vi "display_michelle_visjitter_adj.vi"() -> ()   [LabVIEW 2019]
uses:
  <vilib>/Analysis/Matrix/Datatypes/RealMatrix.ctl
  <vilib>/Utility/file.llb/Write Delimited Spreadsheet (DBL).vi
  <vilib>/Analysis/Matrix/NI_Matrix.lvlib
panel:
  in  "Stop":bool
  out "Num trials":u32=204
  out "ISI Time":dbl
  out "Stim TS":dbl
  out "Output":dbl[][](array[numeric])
  out "Output frame":T1
  out "Array temp1":T1
  out "Elapsed Time":dbl
  out "Display":bool=TRUE
  out "Trial":u32=1
  out "reward":dbl[](array[numeric])
  out "stim_id":dbl[](array[numeric])
  out "stim_loaded":dbl
  out "Timings":dbl[](array[numeric])
  out "Stimuli Loaded?":bool
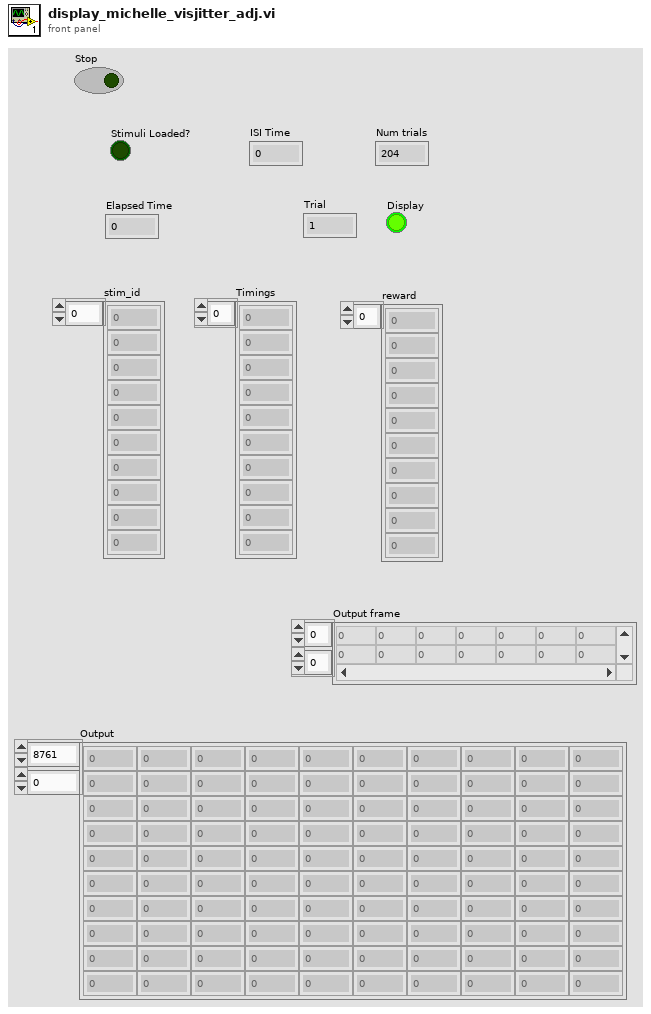
[diagram p1: front panel]
types:
  T1 = typedef "NI_Matrix.lvlib/RealMatrix.ctl" = dbl[][]
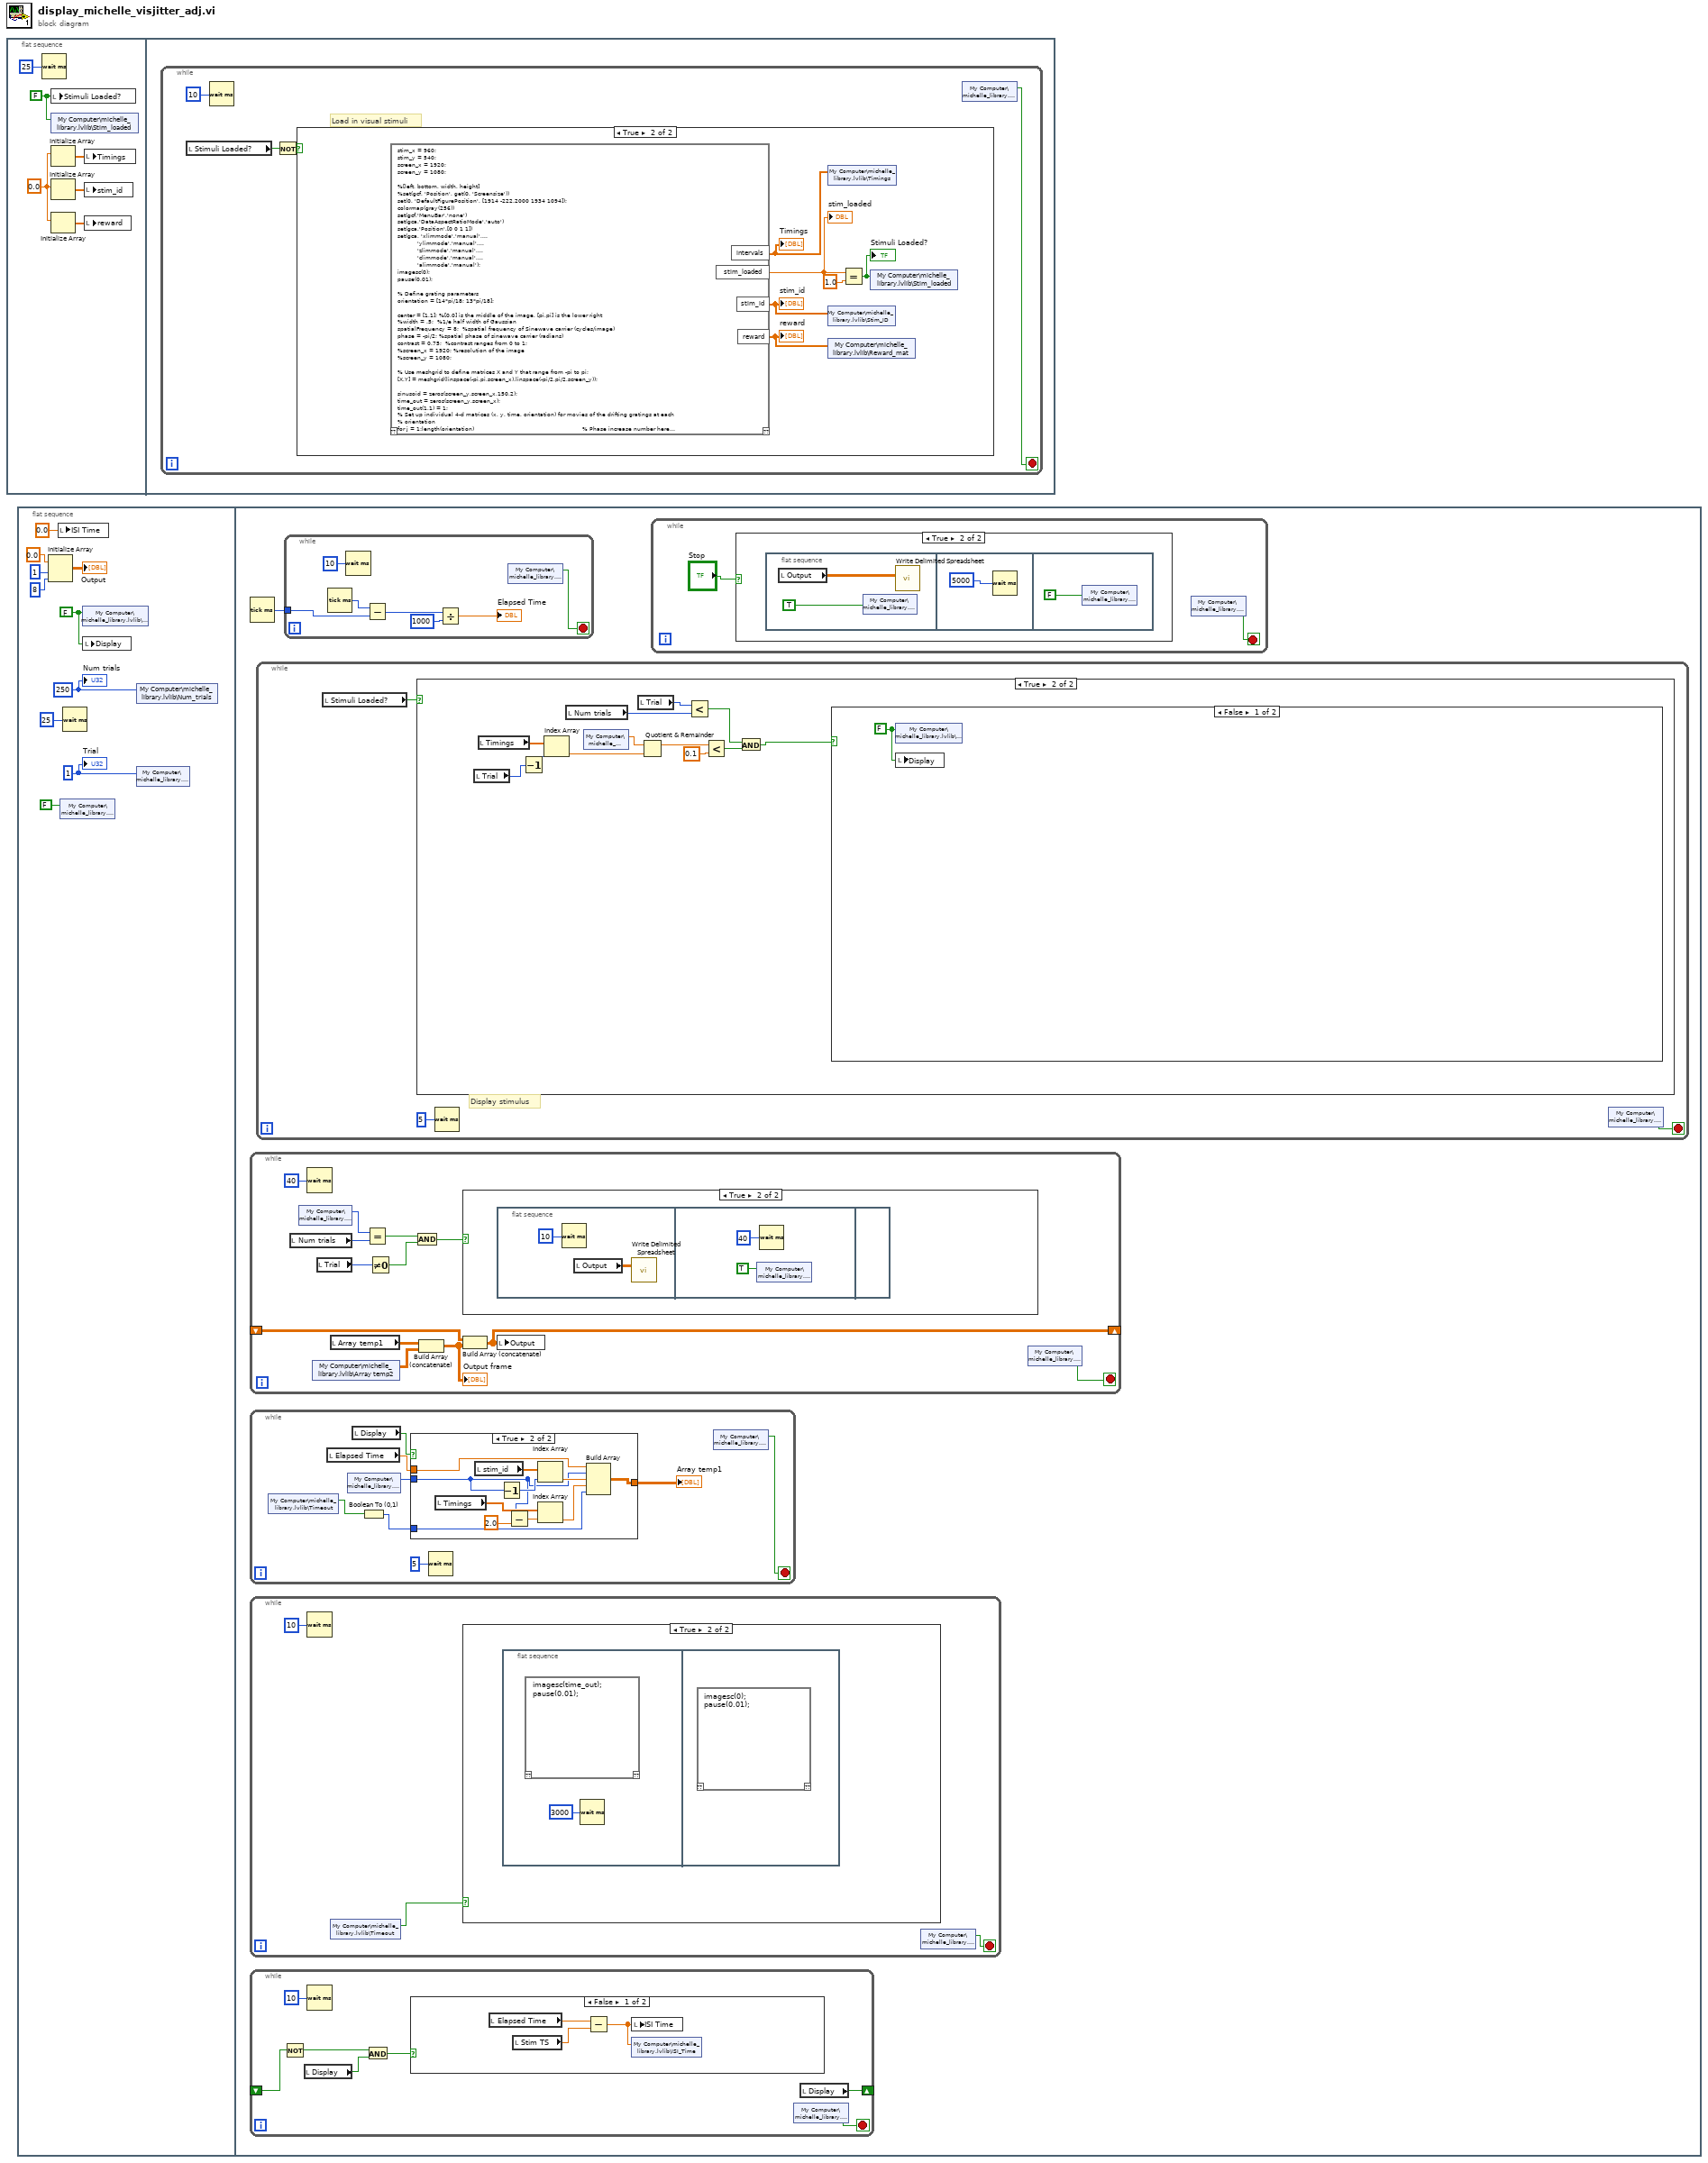
[diagram p0: block diagram]
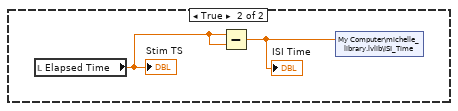
[diagram p5: hidden frame]
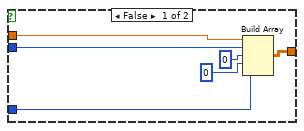
[diagram p6: hidden frame]
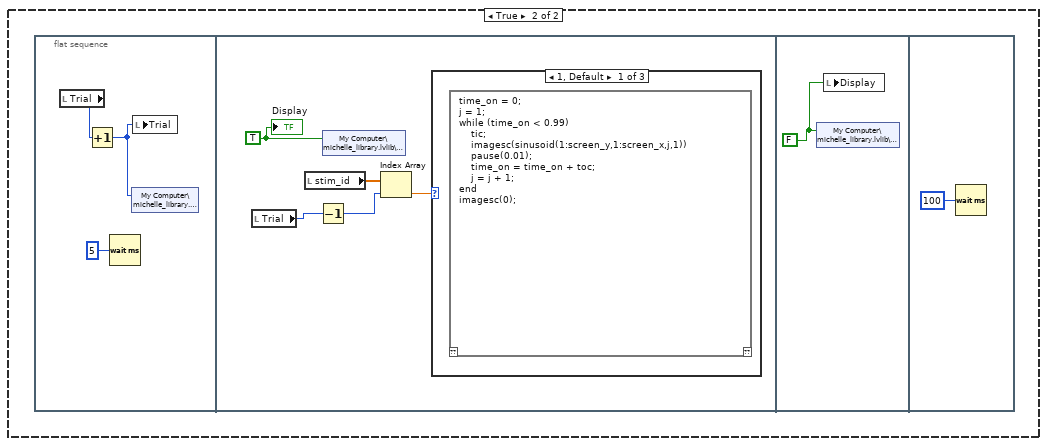
[diagram p9: hidden frame]
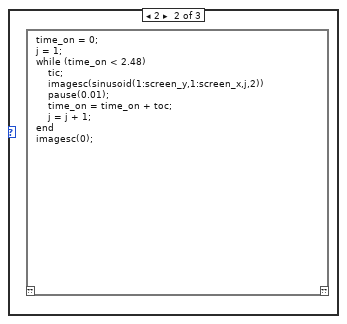
[diagram p10: hidden frame]
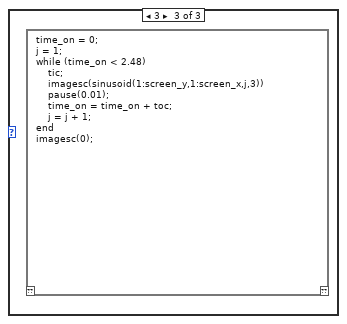
[diagram p11: hidden frame]
diagram:
  n1 = flat-sequence {
    frame #0 {
      w3 = 0.0 ("element")
      w1 = FALSE ("Stimuli Loaded?")
      n2 = Wait (ms)(milliseconds to wait=u32 25) -> ()  [unwired: 1 out]
      n3 = local write "Stimuli Loaded?"(w1) -> ()
      n4 = shared-variable "My Computer\\michelle_library.lvlib\\Stim_loaded"(w1) -> ()  [unwired: 1 in, 1 out]
      n5 = Initialize Array(w3) -> (w5:dbl[])  [unwired: 1 in]
      n6 = Initialize Array(w3) -> (w4:dbl[])  [unwired: 1 in]
      n7 = Initialize Array(w3) -> (w2:dbl[])  [unwired: 1 in]
      n8 = local write "Timings"(w5) -> ()
      n9 = local write "stim_id"(w4) -> ()
      n10 = local write "reward"(w2) -> ()
    }
    frame #1 {
      n11 = while {
        stop <- w9 stop-if-true
        # "Load in visual stimuli"
        n12 = local read "Stimuli Loaded?"() -> (w8:bool)
        n13 = Wait (ms)(milliseconds to wait=u32 10) -> ()  [unwired: 1 out]
        n14 = Not(x=w8) -> (.not. x?=w7:bool)
        n15 = case shown="True" w7 {
          frame False {
          }
          frame True {
            n16 = script code="stim_x = 960;\nstim_y = 540;\nscreen_x = 1920;\nscreen_y = 1080;\n\n%[left, bottom, width, height]\n%set(gcf, 'Position', get(0, 'Screensize'))\nset(0, 'DefaultFigurePosition', [1914 -222.2000 1934 1094]);\ncolormap(gray(256))\nset(gcf,'MenuBar','none')\nset(gca,'DataAspectRatioMode','auto')\nset(gca,'Position',[0 0 1 1])\nset(gca, 'xlimmode','manual',...\n           'ylimmode','manual',...\n           'zlimmode','manual',...\n           'climmode','manual',...\n           'alimmode','manual');\nimagesc(0);\npause(0.01);\n\n% Define grating parameters\norientation = [14*pi/18; 13*pi/18];\n\ncenter = [1,1]; %[0,0] is the middle of the image, [pi,pi] is the lower right\n%width = .5;  %1/e half width of Gaussian\nspatialFrequency = 8;  %spatial frequency of Sinewave carrier (cycles/image)\nphase = -pi/2; %spatial phase of sinewave carrier (radians)\ncontrast = 0.75;  %contrast ranges from 0 to 1;\n%screen_x = 1920; %resolution of the image  \n%screen_y = 1080;\n\n% Use meshgrid to define matrices X and Y that range from -pi to pi;\n[X,Y] = meshgrid(linspace(-pi,pi,screen_x),linspace(-pi/2,pi/2,screen_y));\n\nsinusoid = zeros(screen_y,screen_x,150,2);\ntime_out = zeros(screen_y,screen_x);\ntime_out(1,1) = 1;\n% Set up individual 4-d matrices (x, y, time, orientation) for movies of the drifting gratings at each\n% orientation\nfor j = 1:length(orientation)                                                            % Phase increase number here\n    ramp(1:screen_y,1:screen_x,j) = cos(orientation(j))*(X-center(1)) + sin(orientation(j))*(Y-center(2));     %  |\n    for i = 1:150 %Sets the number of frames to define gratings for                   V\n       sinusoid(1:screen_y,1:screen_x,i,j) = contrast*sin(spatialFrequency*ramp(1:screen_y,1:screen_x,j)-...\n           (phase+(2*pi*(i-1)*(-30)/360))); %Number before '/360' sets the phase increase\n    end\nend\n\n%intervals = [ones(1,41)*10 ones(1,41)*11 ones(1,41)*12 ones(1,41)*13 ones(1,40)*14];\njit = 1.5;\njitter = rand(1,204);\njitter = 2*jit*(jitter- .5);\nITIbase = 3;\nintervals = [ones(1,204)*ITIbase];\nintervals = intervals + jitter;\nstim_id = [ones(1,204)*1];\n%reward = [ones(1,87)*1 ones(1,15)*0 ones(1,87)*1 ones(1,15)*0];\nreward = [ones(1,204)*1];\n\nrand_idx1 = randperm(204);\nrand_idx2 = randperm(204);\nintervals = intervals(rand_idx2);\nstim_id = stim_id(rand_idx2);\nreward = reward(rand_idx2);\n\nstim_loaded = 1;" ("Script Node")() -> ("stim_loaded"=w16:dbl, "intervals"=w11:dbl[], "stim_id"=w12:dbl[], "reward"=w14:dbl[])  [unwired: 1 in, 1 out]
            "stim_loaded" <- w16
            "Timings" <- w11
            "stim_id" <- w12
            "reward" <- w14
            n17 = shared-variable "My Computer\\michelle_library.lvlib\\Timings"(w11) -> ()  [unwired: 1 in, 1 out]
            n18 = shared-variable "My Computer\\michelle_library.lvlib\\Stim_ID"(w12) -> ()  [unwired: 1 in, 1 out]
            n19 = shared-variable "My Computer\\michelle_library.lvlib\\Reward_mat"(w14) -> ()  [unwired: 1 in, 1 out]
            n20 = Equal?(x=w16, y=1.0) -> (x = y?=w13:bool)
            "Stimuli Loaded?" <- w13
            n21 = shared-variable "My Computer\\michelle_library.lvlib\\Stim_loaded"(w13) -> ()  [unwired: 1 in, 1 out]
          }
        }
        n22 = shared-variable "My Computer\\michelle_library.lvlib\\Stop"() -> (w9:bool)  [unwired: 1 in, 1 out]
      }
    }
  }
  n23 = flat-sequence {
    frame #0 {
      w18 = u32 250
      w24 = FALSE ("Display")
      w26 = u32 1 ("Trial")
      n24 = Initialize Array(0.0 ("element"), 1 ("dimension size"), 8 ("dimension size")) -> (→"Output":dbl[][])
      n25 = local write "ISI Time"(0.0 ("ISI Time")) -> ()
      n26 = shared-variable "My Computer\\michelle_library.lvlib\\Stop"(FALSE ("Stop")) -> ()  [unwired: 1 in, 1 out]
      n27 = Wait (ms)(milliseconds to wait=u32 25) -> ()  [unwired: 1 out]
      n28 = shared-variable "My Computer\\michelle_library.lvlib\\Display"(w24) -> ()  [unwired: 1 in, 1 out]
      n29 = local write "Display"(w24) -> ()
      n30 = shared-variable "My Computer\\michelle_library.lvlib\\Num_trials"(w18) -> ()  [unwired: 1 in, 1 out]
      n31 = shared-variable "My Computer\\michelle_library.lvlib\\Trial"(w26) -> ()  [unwired: 1 in, 1 out]
      "Trial" <- w26
      "Num trials" <- w18
    }
    frame #1 {
      n32 = Tick Count (ms)() -> (millisecond timer value=w27:u32)
      n33 = while {
        shift-right: [w91] -> _
        shift-left: _ -> [w92]
        stop <- w94 stop-if-true
        n34 = local read "Num trials"() -> (w86:u32)
        n35 = shared-variable "My Computer\\michelle_library.lvlib\\Trial"() -> (w87:u32)  [unwired: 1 in, 1 out]
        n36 = Wait (ms)(milliseconds to wait=u32 40) -> ()  [unwired: 1 out]
        n37 = shared-variable "My Computer\\michelle_library.lvlib\\Array temp2"() -> (w89:dbl[][])  [unwired: 1 in, 1 out]
        n38 = local read "Trial"() -> (w84:u32)
        n39 = local read "Array temp1"() -> (w90:T1)
        n40 = Equal?(x=w87, y=w86) -> (x = y?=w85:bool)
        n41 = Not Equal To 0?(x=w84) -> (x != 0?=w83:bool)
        n42 = And(x=w85, y=w83) -> (x .and. y?=w82:bool)
        n43 = Build Array (concatenate)(w90, w89) -> (w88:T1)
        "Output frame" <- w88
        n44 = case shown="True" w82 {
          frame False {
          }
          frame True {
            n45 = flat-sequence {
              frame #0 {
                n46 = Wait (ms)(milliseconds to wait=u32 10) -> ()  [unwired: 1 out]
                n47 = local read "Output"() -> (w96:dbl[][])
                n48 = call-poly <vilib>:"Write Delimited Spreadsheet.vi"("2D data"=w96) -> ()  [unwired: 13 in, 2 out]
              }
              frame #1 {
                n49 = shared-variable "My Computer\\michelle_library.lvlib\\Stop"(TRUE) -> ()  [unwired: 1 in, 1 out]
                n50 = Wait (ms)(milliseconds to wait=u32 40) -> ()  [unwired: 1 out]
              }
              frame #2 {
              }
            }
          }
        }
        n51 = Build Array (concatenate) ("Build Matrix")(w92, w88) -> (w91:T1)
        n52 = local write "Output"(w91) -> ()
        n53 = shared-variable "My Computer\\michelle_library.lvlib\\Stop"() -> (w94:bool)  [unwired: 1 in, 1 out]
      }
      n54 = while {
        stop <- w52 stop-if-true
        n55 = shared-variable "My Computer\\michelle_library.lvlib\\Timeout"() -> (w50:bool)  [unwired: 1 in, 1 out]
        n56 = local read "Elapsed Time"() -> (w56:dbl)
        n57 = shared-variable "My Computer\\michelle_library.lvlib\\Trial"() -> (w54:u32)  [unwired: 1 in, 1 out]
        n58 = local read "Display"() -> (w53:bool)
        n59 = Boolean To (0,1)(Boolean=w50) -> (0, 1=w51:i16)
        n60 = case shown="True" w53 {
          tunnel: w54 -> [w62 w65]
          tunnel: w56 -> [w63 w72]
          tunnel: [w61 w73] -> w55
          tunnel: w51 -> [w58 w67]
          frame False {
            n61 = Build Array(w63, w62, u32 0 ("milliseconds to wait"), 0, w58) -> (w61:T1)
          }
          frame True {
            n62 = local read "Timings"() -> (w70:dbl[])
            n63 = local read "stim_id"() -> (w74:dbl[])
            n64 = Decrement(x=w65) -> (x-1=w69:u32)
            n65 = Subtract(x=w65, y=2.0) -> (x-y=w64:dbl)
            n66 = Index Array(array=w74, index=w69) -> (element=w71:dbl)
            n67 = Index Array(array=w70, index=w64) -> (element=w68:dbl)
            n68 = Build Array(w72, w65, w71, w68, w67) -> (w73:T1)
          }
        }
        "Array temp1" <- w55
        n69 = Wait (ms)(milliseconds to wait=u32 5) -> ()  [unwired: 1 out]
        n70 = shared-variable "My Computer\\michelle_library.lvlib\\Stop"() -> (w52:bool)  [unwired: 1 in, 1 out]
      }
      n71 = while {
        stop <- w36 stop-if-true
        n72 = Wait (ms)(milliseconds to wait=u32 10) -> ()  [unwired: 1 out]
        n73 = shared-variable "My Computer\\michelle_library.lvlib\\Timeout"() -> (w34:bool)  [unwired: 1 in, 1 out]
        n74 = case shown="True" w34 {
          frame False {
          }
          frame True {
            n75 = flat-sequence {
              frame #0 {
                n76 = script code="imagesc(time_out);\npause(0.01);"() -> ()  [unwired: 1 in, 1 out]
                n77 = Wait (ms)(milliseconds to wait=u32 3000) -> ()  [unwired: 1 out]
              }
              frame #1 {
                n78 = script code="imagesc(0);\npause(0.01);"() -> ()  [unwired: 1 in, 1 out]
              }
            }
          }
        }
        n79 = shared-variable "My Computer\\michelle_library.lvlib\\Stop"() -> (w36:bool)  [unwired: 1 in, 1 out]
      }
      n80 = while {
        shift-right: [w42] -> _
        shift-left: _ -> [w41]
        stop <- w44 stop-if-true
        n81 = Not(x=w41) -> (.not. x?=w40:bool)
        n82 = local read "Display"() -> (w39:bool)
        n83 = Wait (ms)(milliseconds to wait=u32 10) -> ()  [unwired: 1 out]
        n84 = And(x=w40, y=w39) -> (x .and. y?=w38:bool)
        n85 = case shown="False" w38 {
          frame False {
            n86 = local read "Elapsed Time"() -> (w45:dbl)
            n87 = local read "Stim TS"() -> (w47:dbl)
            n88 = Subtract(x=w45, y=w47) -> (x-y=w46:dbl)
            n89 = local write "ISI Time"(w46) -> ()
            n90 = shared-variable "My Computer\\michelle_library.lvlib\\ISI_Time"(w46) -> ()  [unwired: 1 in, 1 out]
          }
          frame True {
            n91 = local read "Elapsed Time"() -> (w48:dbl)
            "Stim TS" <- w48
            n92 = Subtract(x=w48, y=w48) -> (x-y=w49:dbl)
            "ISI Time" <- w49
            n93 = shared-variable "My Computer\\michelle_library.lvlib\\ISI_Time"(w49) -> ()  [unwired: 1 in, 1 out]
          }
        }
        n94 = shared-variable "My Computer\\michelle_library.lvlib\\Stop"() -> (w44:bool)  [unwired: 1 in, 1 out]
        n95 = local read "Display"() -> (w42:bool)
      }
      n96 = while {
        stop <- w100 stop-if-true
        # "Display stimulus"
        n97 = local read "Stimuli Loaded?"() -> (w99:bool)
        n98 = case shown="True" w99 {
          frame False {
          }
          frame True {
            n99 = local read "Trial"() -> (w102:u32)
            n100 = local read "Timings"() -> (w111:dbl[])
            n101 = Decrement(x=w102) -> (x-1=w103:u32)
            n102 = Index Array(array=w111, index=w103) -> (element=w110:dbl)
            n103 = local read "Num trials"() -> (w106:u32)
            n104 = shared-variable "My Computer\\michelle_library.lvlib\\ISI"() -> (w105:dbl)  [unwired: 1 in, 1 out]
            n105 = local read "Trial"() -> (w109:u32)
            n106 = Quotient & Remainder(x=w105, y=w110) -> (x-y*floor(x/y)=w113:dbl)  [unwired: 1 out]
            n107 = Less?(x=w109, y=w106) -> (x < y?=w108:bool)
            n108 = Less?(x=w113, y=0.1) -> (x < y?=w107:bool)
            n109 = And(x=w108, y=w107) -> (x .and. y?=w104:bool)
            n110 = case shown="False" w104 {
              frame False {
                w114 = FALSE ("Display")
                n111 = shared-variable "My Computer\\michelle_library.lvlib\\Display"(w114) -> ()  [unwired: 1 in, 1 out]
                n112 = local write "Display"(w114) -> ()
              }
              frame True {
                n113 = flat-sequence {
                  frame #0 {
                    n114 = local read "Trial"() -> (w117:u32)
                    n115 = Increment(x=w117) -> (x+1=w116:u32)
                    n116 = Wait (ms)(milliseconds to wait=u32 5) -> ()  [unwired: 1 out]
                    n117 = shared-variable "My Computer\\michelle_library.lvlib\\Trial"(w116) -> ()  [unwired: 1 in, 1 out]
                    n118 = local write "Trial"(w116) -> ()
                  }
                  frame #1 {
                    w121 = TRUE ("Boolean")
                    n119 = local read "Trial"() -> (w119:u32)
                    n120 = local read "stim_id"() -> (w122:dbl[])
                    n121 = Decrement(x=w119) -> (x-1=w118:u32)
                    n122 = shared-variable "My Computer\\michelle_library.lvlib\\Display"(w121) -> ()  [unwired: 1 in, 1 out]
                    n123 = Index Array(array=w122, index=w118) -> (element=w120:dbl)
                    n124 = case shown="1, Default" w120 {
                      frame 1, Default {
                        n125 = script code="time_on = 0;\nj = 1;\nwhile (time_on < 0.99)\n    tic;\n    imagesc(sinusoid(1:screen_y,1:screen_x,j,1))\n    pause(0.01);\n    time_on = time_on + toc;\n    j = j + 1;\nend\nimagesc(0);"() -> ()  [unwired: 1 in, 1 out]
                      }
                      frame 2 {
                        n126 = script code="time_on = 0;\nj = 1;\nwhile (time_on < 2.48)\n    tic;\n    imagesc(sinusoid(1:screen_y,1:screen_x,j,2))\n    pause(0.01);\n    time_on = time_on + toc;\n    j = j + 1;\nend\nimagesc(0);"() -> ()  [unwired: 1 in, 1 out]
                      }
                      frame 3 {
                        n127 = script code="time_on = 0;\nj = 1;\nwhile (time_on < 2.48)\n    tic;\n    imagesc(sinusoid(1:screen_y,1:screen_x,j,3))\n    pause(0.01);\n    time_on = time_on + toc;\n    j = j + 1;\nend\nimagesc(0);"() -> ()  [unwired: 1 in, 1 out]
                      }
                    }
                    "Display" <- w121
                  }
                  frame #2 {
                    w123 = FALSE ("Display")
                    n128 = shared-variable "My Computer\\michelle_library.lvlib\\Display"(w123) -> ()  [unwired: 1 in, 1 out]
                    n129 = local write "Display"(w123) -> ()
                  }
                  frame #3 {
                    n130 = Wait (ms)(milliseconds to wait=u32 100) -> ()  [unwired: 1 out]
                  }
                }
              }
            }
          }
        }
        n131 = Wait (ms)(milliseconds to wait=u32 5) -> ()  [unwired: 1 out]
        n132 = shared-variable "My Computer\\michelle_library.lvlib\\Stop"() -> (w100:bool)  [unwired: 1 in, 1 out]
      }
      n133 = while {
        tunnel: w27 -> [w78]
        stop <- w75 stop-if-true
        n134 = Tick Count (ms)() -> (millisecond timer value=w79:u32)
        n135 = Wait (ms)(milliseconds to wait=u32 10) -> ()  [unwired: 1 out]
        n136 = Subtract(x=w79, y=w78) -> (x-y=w76:u32)
        n137 = Divide(x=w76, y=u32 1000) -> (x/y=→"Elapsed Time":dbl)
        n138 = shared-variable "My Computer\\michelle_library.lvlib\\Stop"() -> (w75:bool)  [unwired: 1 in, 1 out]
      }
      n139 = while {
        stop <- w28 stop-if-true
        n140 = case shown="True" "Stop" {
          frame False {
          }
          frame True {
            n141 = flat-sequence {
              frame #0 {
                n142 = local read "Output"() -> (w31:dbl[][])
                n143 = shared-variable "My Computer\\michelle_library.lvlib\\Stop"(TRUE ("Stop")) -> ()  [unwired: 1 in, 1 out]
                n144 = call-poly <vilib>:"Write Delimited Spreadsheet.vi"("2D data"=w31) -> ()  [unwired: 13 in, 2 out]
              }
              frame #1 {
                n145 = Wait (ms)(milliseconds to wait=u32 5000) -> ()  [unwired: 1 out]
              }
              frame #2 {
                n146 = shared-variable "My Computer\\michelle_library.lvlib\\Stop"(FALSE ("Stop")) -> ()  [unwired: 1 in, 1 out]
              }
            }
          }
        }
        n147 = shared-variable "My Computer\\michelle_library.lvlib\\Stop"() -> (w28:bool)  [unwired: 1 in, 1 out]
      }
    }
  }
